vi "ReportGenerator.Graph.vi"(7 "Graph reference":refnum<vi>, 8 "error in (no error)":errorcluster, 9 "Font":T1, 10 "Graph name":string, 11 "NI_report in":refnum<class "NI_report.lvclass">) -> (0 "error out":errorcluster, 3 "NI_report out":refnum<class "NI_report.lvclass">)   [LabVIEW 2019, in "Tools.lvlib"]
uses:
  <vilib>/Utility/NIReport.llb/NI_report.lvclass
  <vilib>/Utility/NIReport.llb/Append Report Text (str wrap).vi
  Tools.lvlib
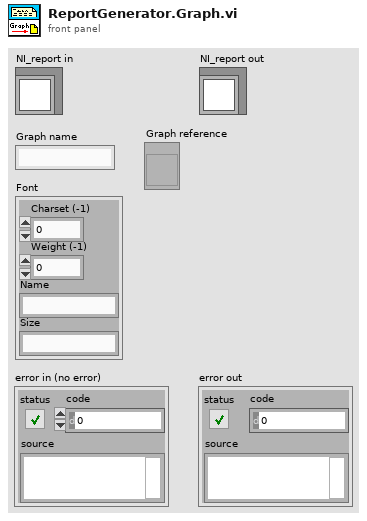
[diagram p1: front panel]
types:
  T1 = cluster{"Charset (-1)":i16, "Weight (-1)":i16, "Name":string, "Size":string}
  T2 = cluster{"Italic":enum16{"Italic Unchanged", "Italic On", "Italic Off"}, "Strike Through":enum16{"Strike Through Unchanged", "Strike Through On", "Strike Through Off"}, "Underline":enum16{"Underline Unchanged", "Underline On", "Underline Off"}, "Bold":enum16{"Bold Unchanged", "Bold On", "Bold Off"}}
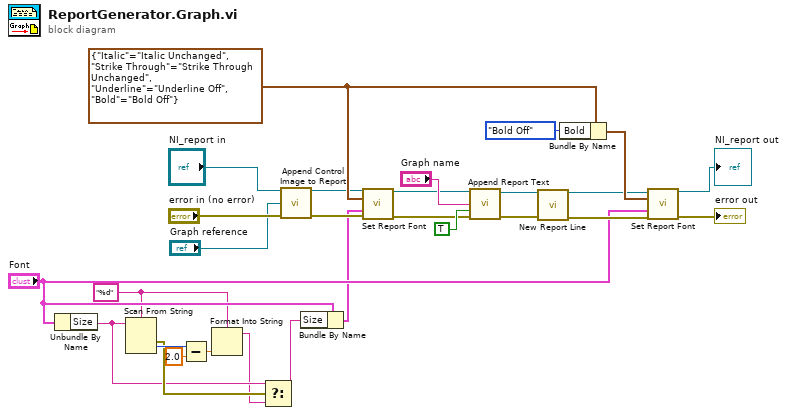
[diagram p0: block diagram]
diagram:
  w1 = "%d" ("format string")
  w24 = T2 {"Italic"=enum."Italic Unchanged", "Strike Through"=enum."Strike Through Unchanged", "Underline"=enum."Underline Off", "Bold"=enum."Bold Off"} ("text options")
  n1 = Unbundle By Name("Font") -> ("Size"=w7:string)
  n2 = Scan From String(format string=w1, input string=w7) -> (error out=w8:errorcluster, output 1=w10:i32)  [unwired: 3 in, 2 out]
  n3 = Subtract(x=w10, y=2.0 ("x")) -> (x-y=w9:dbl)
  n4 = Format Into String(format string=w1, w9) -> (resulting string=w6:string)  [unwired: 2 in, 1 out]
  n5 = Select(t=w7, s=w8, f=w6) -> (s? t:f=w5:string)
  n6 = call-dynamic "Append Control Image to Report.vi"("report in"="NI_report in", "ctrl reference"="Graph reference", "error in (no error)"="error in (no error)") -> ("report out"=w15:refnum<class "NI_report.lvclass">, "error out"=w13:errorcluster)  [unwired: 9 in, 2 out]
  n7 = Bundle By Name(cluster="Font", "Size"=w5) -> (w3:T1)
  n8 = call-dynamic "Set Report Font.vi"("report in"=w15, "text options"=w24, "font settings"=w3, "error in (no error)"=w13) -> ("report out"=w21:refnum<class "NI_report.lvclass">, "error out"=w22:errorcluster)  [unwired: 9 in, 1 out]
  n9 = call-poly <vilib>:"Append Report Text.vi"("report in"=w21, "text"="Graph name", "append on new line? (F)"=TRUE, "error in (no error)"=w22) -> ("report out"=w20:refnum<class "NI_report.lvclass">, "error out"=w19:errorcluster)  [unwired: 8 in, 2 out]
  n10 = call-dynamic "New Report Line.vi"("report in"=w20, "error in (no error)"=w19) -> ("report out"=w17:refnum<class "NI_report.lvclass">, "error out"=w18:errorcluster)  [unwired: 12 in]
  n11 = Bundle By Name(cluster=w24, "Bold"=enum16{"Bold Unchanged", "Bold On", "Bold Off"}."Bold Off") -> (w25:T2)
  n12 = call-dynamic "Set Report Font.vi"("report in"=w17, "text options"=w25, "font settings"="Font", "error in (no error)"=w18) -> ("report out"=→"NI_report out":refnum<class "NI_report.lvclass">, "error out"=→"error out":errorcluster)  [unwired: 9 in, 1 out]
